vi "Destroy Registry.vi"(8 "error in (no error)":errorcluster, 11 "Registry in":refnum<class "Registry.lvclass">) -> (0 "error out":errorcluster, 1 "Values":variant[](array[variant]) caption="Data", 2 "Keys":string[](array[string]) caption="Names", 3 "Registry out":refnum<class "Registry.lvclass">)   [LabVIEW 2020, in "BCI-1553 API.lvlib" / "Registry.lvlib" / "Registry.lvclass"]
doc: "Destroys the Registry and returns all the current contents of the Registry."
uses:
  Registry.lvclass
  Registry.lvclass/Registry.ctl
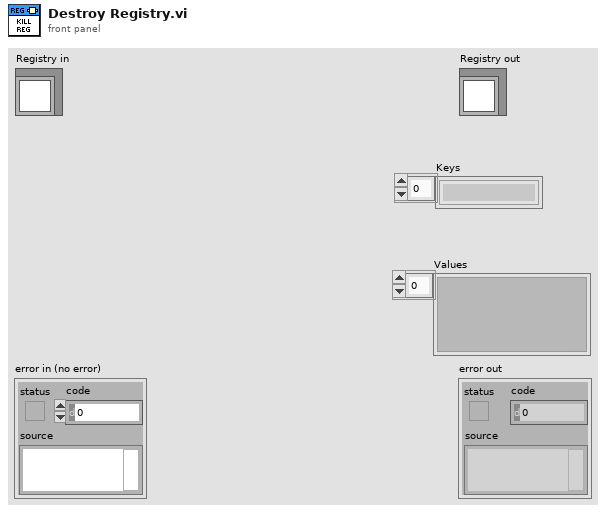
[diagram p1: front panel]
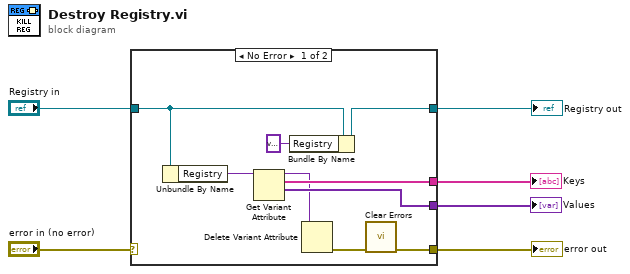
[diagram p0: block diagram]
diagram:
  n1 = case shown="No Error" "error in (no error)" {
    selector: "error in (no error)" -> [_ w17]
    tunnel: [w15 w17] -> w5
    tunnel: [w7 w16] -> w3
    tunnel: "Registry in" -> [w8 w16]
    tunnel: [w14 _] -> w2
    tunnel: [w13 _] -> w1
    frame No Error {
      n2 = Unbundle By Name(w8) -> ("Registry"=w12:variant)
      n3 = Get Variant Attribute(Variant=w12) -> (duplicate Variant=w11:variant, names=w14:string[], values=w13:variant[])  [unwired: 3 in, 1 out]
      n4 = Bundle By Name(cluster=w8, "Registry"=variant) -> (w7:refnum<class "Registry.lvclass">)
      n5 = Delete Variant Attribute(7:w11) -> (0:w10:errorcluster)  [unwired: 2 in, 2 out]
      n6 = call <vilib>:"Clear Errors.vi"("error in (no error)"=w10) -> ("error out"=w15:errorcluster)  [unwired: 5 in, 1 out]
    }
    frame Error {
    }
  }
  "error out" <- w5
  "Registry out" <- w3
  "Keys" <- w2
  "Values" <- w1
